vi "Bertta_v09_1.vi"() -> ()   [LabVIEW 2015]
panel:
  out "element":bool
  out "Started:":string
  in  "SHUTDOWN":bool
  in  "MASTER CONTROL":bool
  in  "Tab Control":T1(tab)
  in  "Read Seq":bool
  in  "Save Seq":bool
  in  "Configuration file":path=path "C:/Users/shresplab/Desktop/BerttaConfiguration.lvm" caption="Filename"
  in  "OK Button 2":bool
  out "Boolean":bool
  in  "User (initials)":string
  in  "Project name":string
  in  "Description":string
  out "Output file":string
  out "Sensor OK 6":bool
  out "Sensor OK 5":bool
  out "Sensor OK 4":bool
  out "Sensor OK 3":bool
  in  "OK Button":bool
  in  "Add comment":string
  out "PUMP 1":bool
  out "Target amount":dbl
  out "Scale weight":dbl
  out "Amount now":dbl
  out "Flow rate":dbl
  out "Time to target":dbl format="%<%H:%M:%S>t"
  out "Current step":dbl
  out "Target amount":dbl
  out "Amount now":dbl
  out "Tr":dbl
  out "Tj in":dbl
  out "Tj out":dbl
  out "T set":dbl
  out "Current step":i32
  out "RPM":dbl
  out "Torque 2":dbl
  out "Waveform Chart 5":dynamicdata(graph)
  out "Waveform Chart 6":dynamicdata(graph)
  out "Waveform Chart 7":dynamicdata(graph)
  out "Amount now":dbl
  out "Target amount":dbl
  out "Current step":dbl
  out "Time to target":dbl format="%<%H:%M:%S>t"
  out "Flow rate":dbl
  out "Amount now":dbl
  out "Scale weight":dbl
  out "Target amount":dbl
  out "PUMP 2":bool
  in  "Tab Control 2":T2(tab)
  out "Waveform Chart 3":dynamicdata(graph)
  out "Waveform Chart 8":dynamicdata(graph)
  out "Waveform Chart 11":dynamicdata(graph)
  out "Waveform Chart 9":dynamicdata(graph)
  out "Table":string[][](table)=[["14.8.2017 18.06.59", "0,000000", "417,670000", "-0,150000", "1,000000", "22,220000", "23,366837", "23,574959", "23,985852", "23,690000", "240,000000", "4,000000", "0,000000", "397,000000", "-397,000000", "1,000000"], ["14.8.2017 18.07.06", "0,000000", "417,640000", "-0,120000", "1,000000", "22,220000", "23,763115", "23,906257", "23,985694", "23,680000", "240,000000", "4,000000", "0,000000", "397,000000", "-397,000000", "1,000000"], ["14.8.2017 18.07.13", "0,000000", "417,640000", "-0,120000", "1,000000", "22,220000", "23,965922", "24,013440", "23,984906", "23,670000", "240,000000", "4,100000", "3,000000", "397,000000", "-397,000000", "1,000000"], ["14.8.2017 18.07.21", "0,000000", "417,640000", "-0,120000", "1,000000", "22,220000", "23,943860", "23,900110", "23,987113", "23,670000", "240,000000", "4,000000", "0,000000", "397,000000", "-397,000000", "1,000000"], ["14.8.2017 18.07.28", "0,000000", "417,640000", "-0,120000", "1,000000", "22,220000", "23,736328", "23,600018", "23,989004", "23,660000", "240,000000", "4,000000", "0,000000", "397,000000", "-397,000000", "1,000000"], ["14.8.2017 18.07.36", "0,000000", "417,640000", "-0,120000", "1,000000", "22,220000", "23,480910", "23,324538", "23,991053", "23,660000", "240,000000", "4,000000", "0,000000", "397,000000", "-397,000000", "1,000000"], ["14.8.2017 18.07.43", "0,000000", "417,640000", "-0,120000", "2,000000", "22,220000", "23,195579", "23,008270", "23,999093", "23,650000", "240,000000", "4,000000", "0,000000", "397,000000", "-397,000000", "1,000000"], ["14.8.2017 18.07.51", "0,000000", "417,650000", "-417,650000", "1,000000", "22,220000", "22,862541", "22,649021", "24,003979", "23,650000", "240,000000", "4,000000", "0,000000", "397,000000", "-397,000000", "2,000000"], ["14.8.2017 18.07.58", "0,000000", "417,640000", "0,010000", "1,000000", "22,220000", "22,541353", "22,354878", "24,005398", "23,650000", "240,000000", "4,000000", "0,000000", "397,000000", "-397,000000", "1,000000"], ["14.8.2017 18.08.06", "0,000000", "417,640000", "0,010000", "1,000000", "22,220000", "22,347931", "22,253738", "24,007605", "23,640000", "240,000000", "4,100000", "0,000000", "397,000000", "-397,000000", "1,000000"], ["14.8.2017 18.08.13", "0,000000", "417,640000", "0,010000", "1,000000", "22,220000", "22,329030", "22,302102", "24,006028", "23,640000", "240,000000", "4,000000", "0,000000", "395,820000", "-395,820000", "1,000000"], ["14.8.2017 18.08.20", "0,000000", "417,640000", "0,010000", "1,000000", "22,220000", "22,466849", "22,511320", "24,002403", "23,630000", "240,000000", "4,000000", "0,000000", "395,830000", "-0,010000", "1,000000"], ["14.8.2017 18.08.28", "0,000000", "417,640000", "0,010000", "1,000000", "22,220000", "22,707062", "22,835101", "24,000984", "23,620000", "240,000000", "4,000000", "0,000000", "395,830000", "-0,010000", "1,000000"], ["14.8.2017 18.08.35", "0,000000", "417,640000", "0,010000", "1,000000", "22,220000", "23,054104", "23,232979", "24,001299", "23,600000", "240,000000", "4,000000", "0,000000", "395,830000", "-0,010000", "1,000000"], ["14.8.2017 18.08.43", "0,000000", "417,640000", "0,010000", "1,000000", "22,220000", "23,412371", "23,522793", "24,002560", "23,590000", "240,000000", "4,000000", "0,000000", "395,820000", "0,000000", "1,000000"], ["14.8.2017 18.08.51", "0,000000", "417,640000", "0,010000", "1,000000", "22,220000", "23,596247", "23,656125", "24,003821", "23,580000", "240,000000", "4,000000", "0,000000", "395,820000", "0,000000", "1,000000"]]
  in  "T ext / T ext 2":enum32{"External 1", "External 2"}(radio)
  out "Sensor OK":bool
  in  "T fail":dbl=20.0
  out "Boolean 12":bool
  out "Boolean 7":bool
  out "Boolean 6":bool
  out "Boolean 5":bool
  out "Boolean 4":bool
  in  "?":bool
  in  "T manual setpoint":dbl=20.0
  in  "Lauda port":dbl=9.0
  in  "Manual select":enum32{"Tr", "Tj"}(radio)
  in  "TempSeq":dbl[][](array[numeric])=[[20.0, 40.0, 1.0, 30.0], [40.0, 50.0, 1.0, 30.0], [50.0, 20.0, 1.0, 30.0], [20.0, 20.0, 0.0, 20.0], [20.0, 20.0, 0.0, 20.0], [20.0, 20.0, 1000.0, 20.0]]
  out "T control":dbl
  out "Tr":dbl
  out "Tj in":dbl
  out "Tj out":dbl
  out "DT":dbl
  out "Elapsed":i32 format="%<%H:%M:%S>T"
  in  "PAUSE":bool
  out "Boolean 19":bool
  in  "Reset":bool
  in  "Treshold (Tset)":dbl=1.0
  in  "Tmax":dbl=199.0
  in  "Tmin":dbl=20.0
  out "Waveform Chart":dynamicdata(graph)
  out "T external 2":dbl
  in  "Xe":dbl=1.0
  in  "Ring":u16(ring) items=["SCALE 1", "SCALE 2", "SCALE 3"]
  out "Port":i32=10
  in  "Radio Buttons":enum32{"Reglo Digital", "Reglo Analog", "PAM"}(radio)=enum."Reglo Analog"
  out "Speed":dbl
  out "mA":dbl format="%#_2g"
  in  "Port":i32=14
  out "RPM":dbl format="%#_2g"
  out "Led10":bool
  out "Led9":bool
  out "Led8":bool
  out "Led7":bool
  out "Led6":bool
  out "Led5":bool
  out "Led4":bool
  out "Led3":bool
  out "Led2":bool
  out "Led1":bool
  in  "PumpSeq":dbl[][](array[numeric])=[[3.0, 3.0, 7.0], [2.0, 2.0, 2.0], [4.0, 2.0, 100.0], [0.0, 0.0, 0.0], [0.0, 0.0, 0.0], [0.0, 0.0, 0.0], [0.0, 0.0, 0.0], [0.0, 0.0, 0.0], [0.0, 0.0, 0.0], [0.0, 0.0, 0.0], [0.0, 1.0, 0.0]]
  in  "?":bool
  out "Flow rate (g/min)":dbl
  out "Scale reading":dbl
  out "Step amount now":dbl
  out "Time to target":dbl format="%<%H:%M:%S>t"
  in  "Grams / min":dbl
  out "Waveform Chart 2":dynamicdata(graph)
  in  "?":bool
  out "Total amount now":dbl
  out "Total time":dbl
  out "Total amount target":dbl
  out "Led11":bool
  in  "Reset 2":bool
  in  "Bypass select 2":enum32{"Remote", "Manual"}(radio)
  in  "Port":dbl=13.0
  out "RPM":dbl
  out "Torque":dbl
  in  "Set RPM":dbl(slide) scale=0.0..500.0
  out "Waveform Chart 4":dynamicdata(graph)
  out "DAQ 9217 (PT100)":errorcluster
  # "PUMP & SCALE 1"
  # "PUMP & SCALE 2"
  # "STEP"
  # "STEP"
  # "TOTAL"
  # "TOTAL"
  # "Temperature sensor:"
  # "Manual control:"
  # "Tinit     >    Tset       Min. time      Tfail"
  # "Manual control / end of sequence"
  # "Manual control"
  # "Secondary temperature sensor"
  # "Device communication"
  # "Grams    /   min"
  # "End of sequence"
  # "Manual control"
  # "Device communication"
  # "Pump configuration"
  # "Scale configuration"
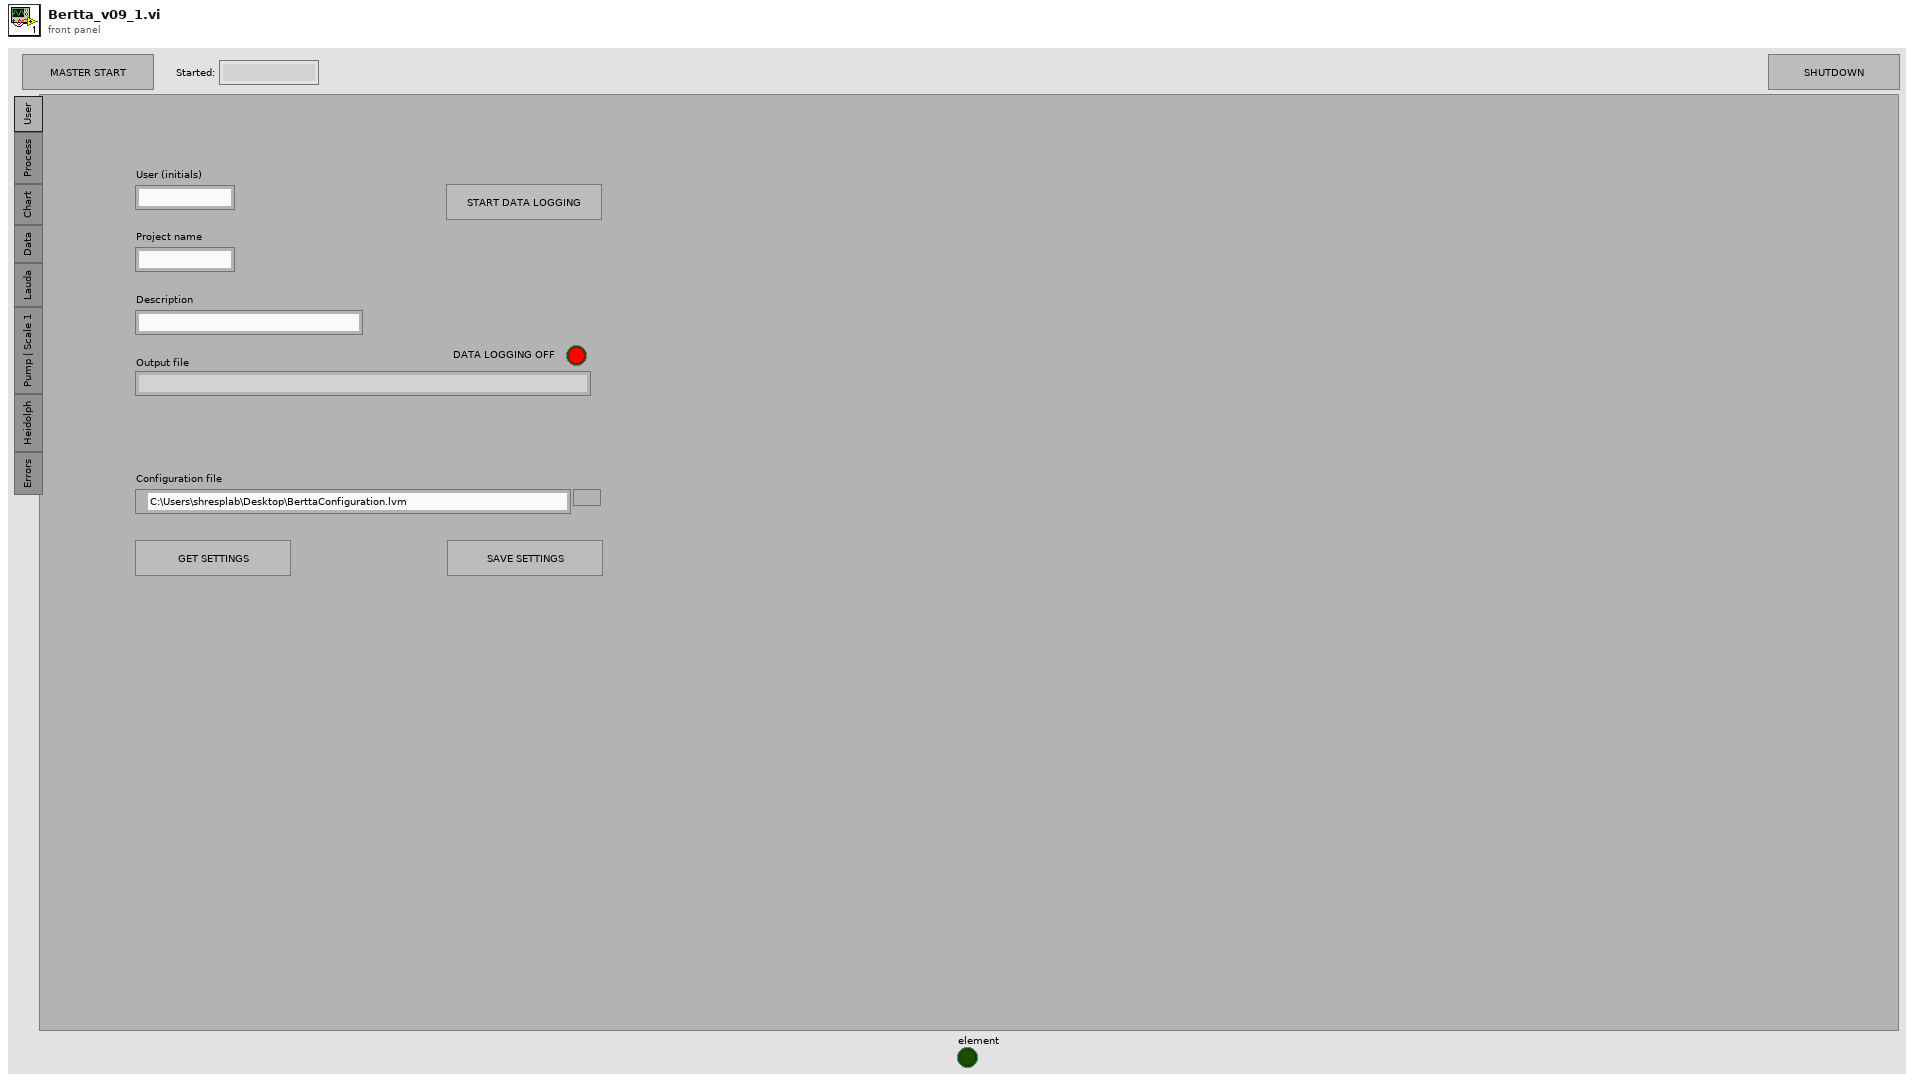
[diagram p1: front panel]
types:
  T1 = enum32{"User", "Process", "Chart", "Data", "Lauda", "Pump | Scale 1", "Heidolph", "Errors"}
  T2 = enum32{"Temperatures", "Scale / Pump 1", "Scale / Pump 2", "RPM / torque"}
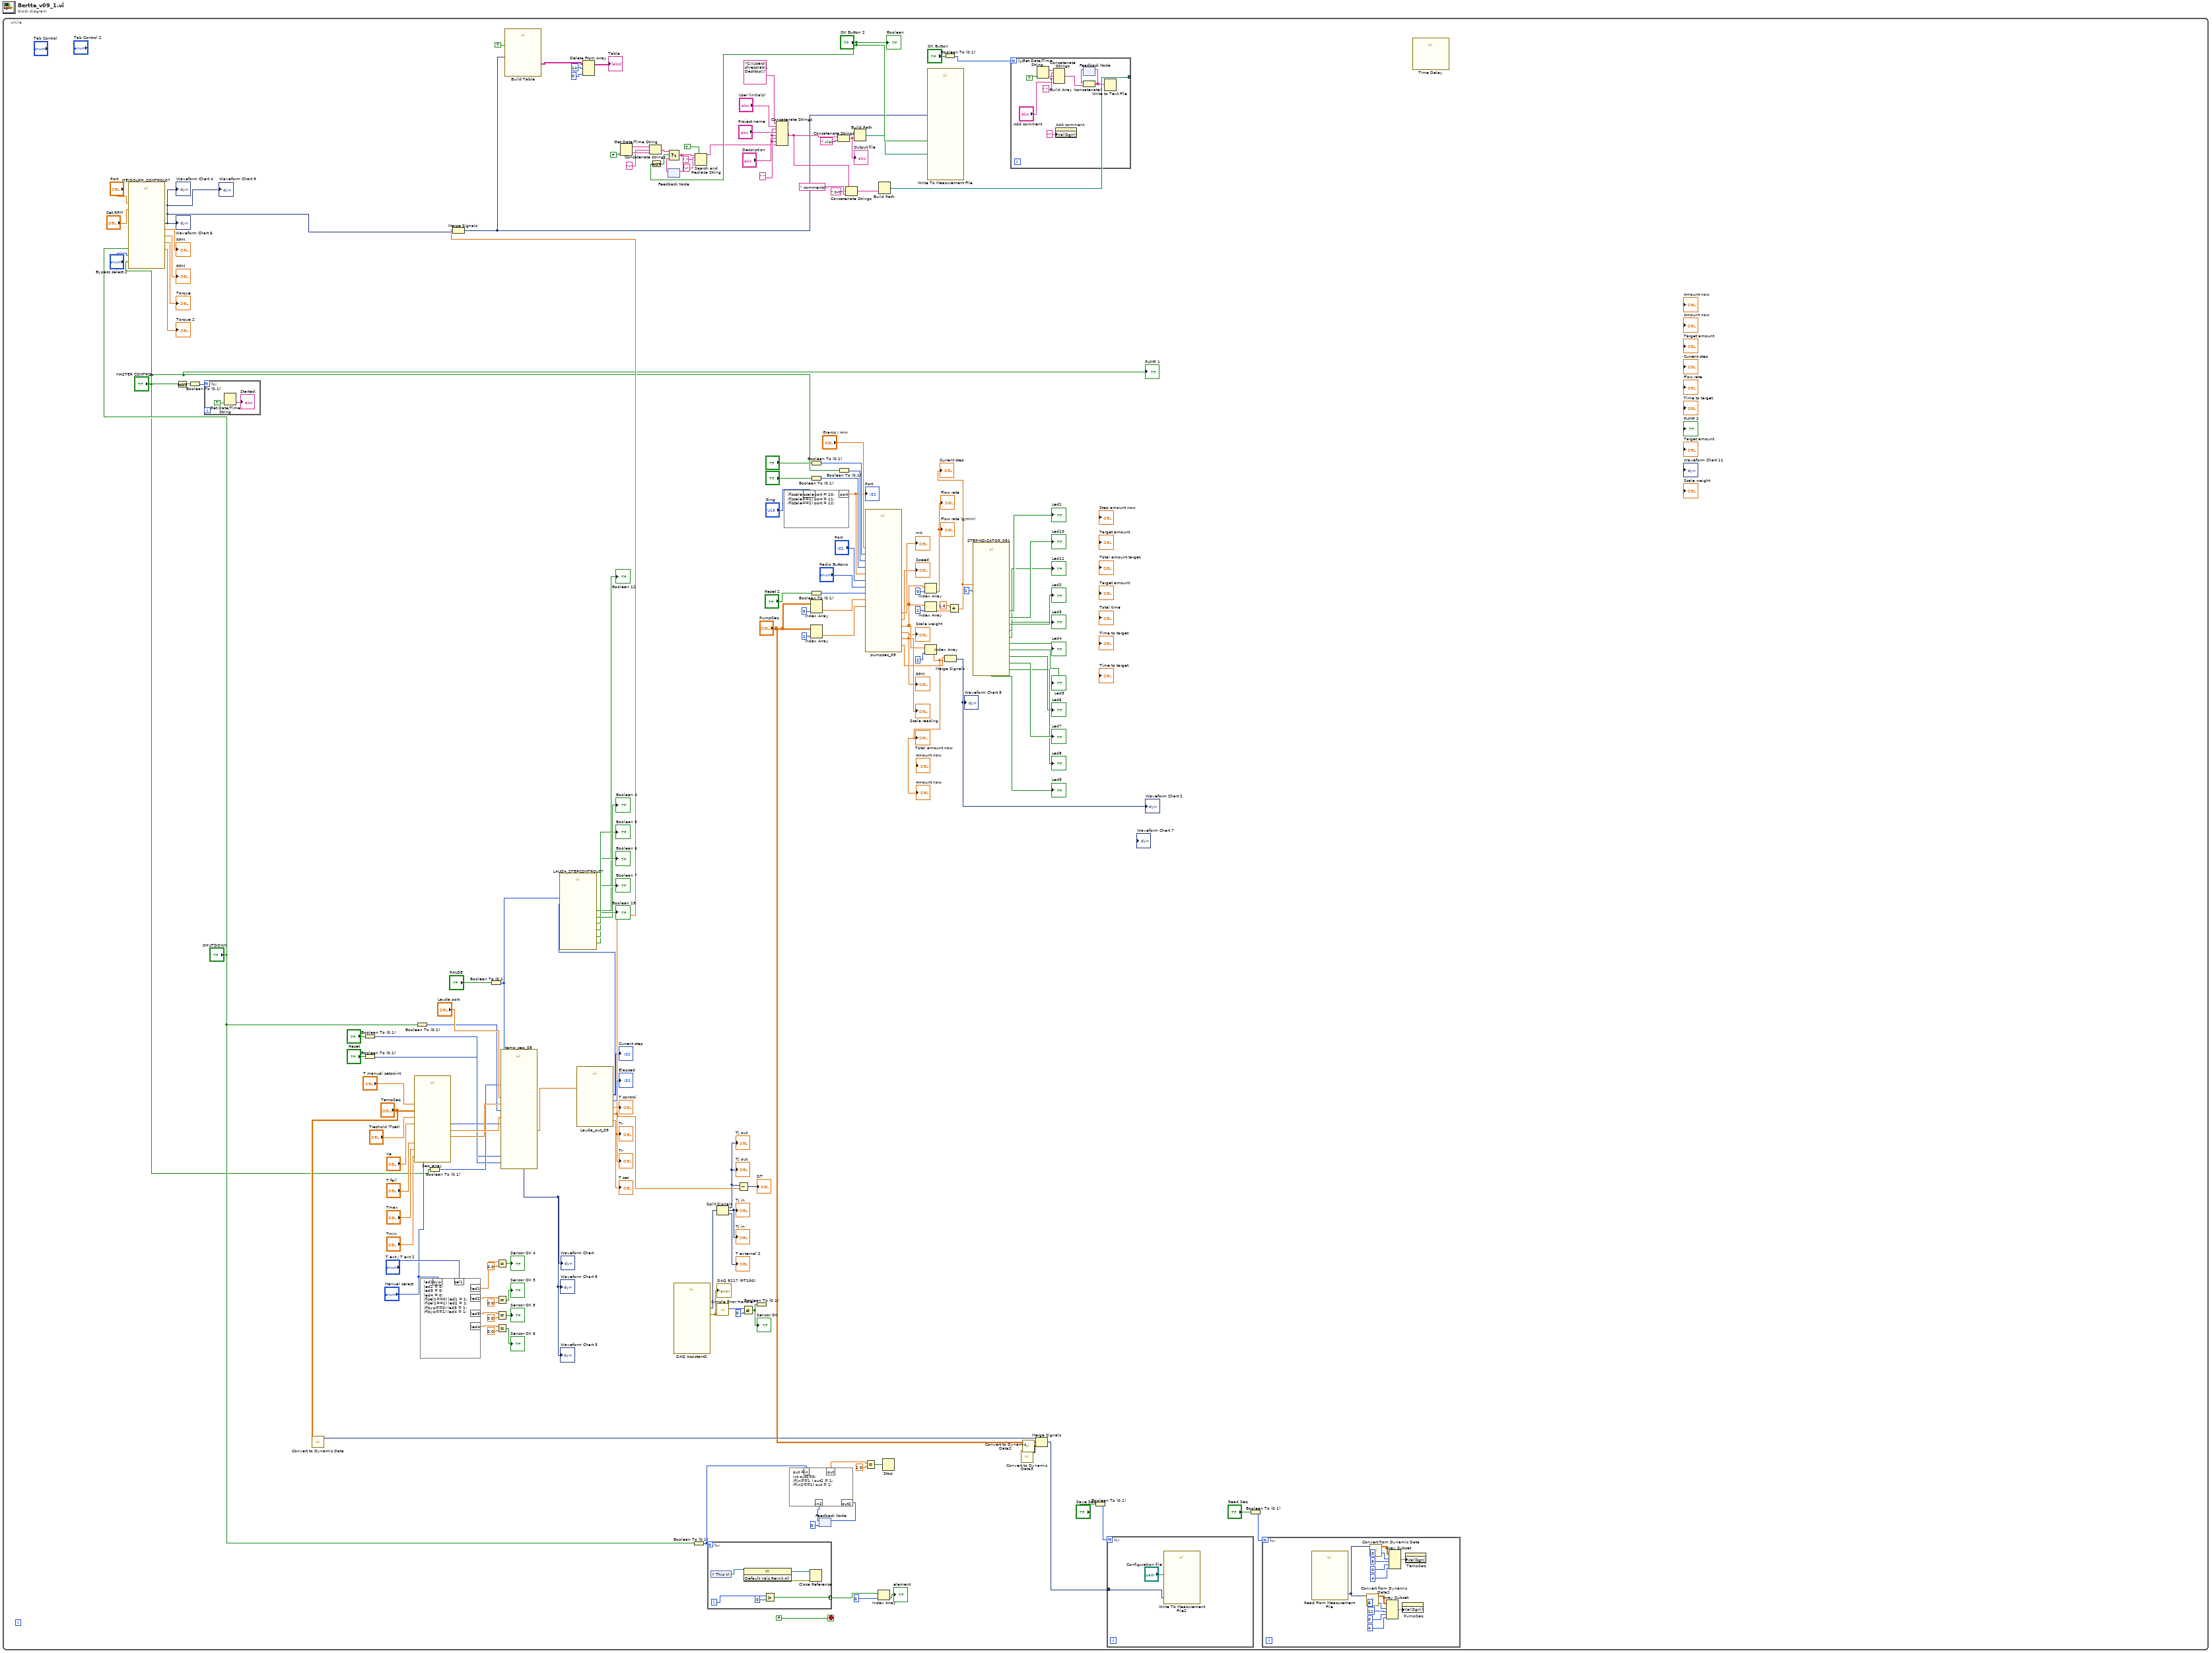
[diagram p0: block diagram]
diagram:
  n1 = while {
    stop <- FALSE stop-if-true
    w146 = " "
    n2 = call "HEIDOLPH_CONTROL07.vi"("master"="MASTER CONTROL", "shutdown"="SHUTDOWN", "Bypass select"="Bypass select 2", "Set RPM"="Set RPM", "Device port"="Port") -> ("Dynamic Data"=w157:dynamicdata, "RPM"=→"RPM":dbl, "RPM 2"=→"RPM":dbl, "Torque"=→"Torque":dbl, "Torque 2"=→"Torque 2":dbl)  [unwired: 2 in]
    "Waveform Chart 4" <- w157
    "Waveform Chart 6" <- w157
    "Waveform Chart 9" <- w157
    n3 = Not(x="MASTER CONTROL") -> (.not. x?=w139:bool)
    n4 = Boolean To (0,1)(Boolean=w139) -> (0, 1=w140:i16)
    n5 = for {
      N: w140 -> [_]
      n6 = Get Date/Time String(want seconds? (F)=TRUE) -> (time string=→"Started:":string)  [unwired: 2 in, 1 out]
    }
    n7 = call "Convert to Dynamic Data"("2D Array"="TempSeq") -> ("Dynamic Data Type"=w136:dynamicdata)  [unwired: 3 in]
    n8 = Boolean To (0,1)(Boolean="Reset") -> (0, 1=w58:i16)
    n9 = Boolean To (0,1)(Boolean="?") -> (0, 1=w60:i16)
    n10 = call "Seq_array.vi"("Tfail_manual"="T fail", "TempSeq in"="TempSeq", "Tmin"="Tmin", "Tmax"="Tmax", "Treshold (Tset)"="Treshold (Tset)", "T manual setpoint"="T manual setpoint", "Xe"="Xe") -> ("TimeParams"=w73:dbl[], "TempParams"=w74:dbl[])  [unwired: 3 in]
    n11 = Boolean To (0,1)(Boolean="SHUTDOWN") -> (0, 1=w69:i16)
    n12 = formula code="led1 = 0;\nled2 = 0;\nled3 = 0;\nled4 = 0;\nif(sel1==0) led1 = 1;\nif(sel1==1) led2 = 1;\nif(byp==0) led3 = 1;\nif(byp==1) led4 = 1;"("sel1"="T ext / T ext 2", "byp"="Manual select") -> ("led1"=w89:dbl, "led2"=w87:dbl, "led3"=w82:dbl, "led4"=w81:dbl)
    n13 = Boolean To (0,1)(Boolean="MASTER CONTROL") -> (0, 1=w68:i16)
    n14 = Boolean To (0,1)(Boolean="PAUSE") -> (0, 1=w64:i16)
    n15 = Equal?(x=w89, y=0.0) -> (x = y?=→"Sensor OK 4":bool)
    n16 = Equal?(x=w87, y=0.0) -> (x = y?=→"Sensor OK 3":bool)
    n17 = Equal?(x=w82, y=0.0) -> (x = y?=→"Sensor OK 5":bool)
    n18 = Equal?(x=w81, y=0.0) -> (x = y?=→"Sensor OK 6":bool)
    n19 = call "temp_seq_09.vi"("master"=w68, "shutdown"=w69, "Tr_orTj"="Manual select", "pause"=w64, "TempParams"=w74, "TimeParams"=w73, "port"="Lauda port", "reset"=w58, "manual"=w60) -> ("params"=w66:dbl[], "Waveform Chart"=→"Waveform Chart 3" →"Waveform Chart" →"Waveform Chart 5":dynamicdata)  [unwired: 3 in, 2 out]
    n20 = call "Lauda_out_09.vi"("params"=w66) -> ("Elapsed"=→"Elapsed":i32, "Tr"=w48:dbl, "Current step"=w47:i32, "T control"=→"T control":dbl, "T set"=→"T set":dbl)  [unwired: 6 in]
    "Tr" <- w48
    "Tr" <- w48
    "Current step" <- w47
    n21 = Merge Signals(w48, w157) -> (w112:dynamicdata)
    n22 = call "Build Table"("Include time data"=TRUE, "Signals"=w112) -> ("Table"=w111:string[][])  [unwired: 3 in, 6 out]
    n23 = call "LAUDA_STEPCONTROL07.vi"("step"=w47, "pause"=w64) -> ("Boolean 13"=→"Boolean 19":bool, "Boolean 6"=→"Boolean 6":bool, "Boolean 5"=→"Boolean 5":bool, "Boolean 4"=→"Boolean 4":bool, "Boolean 7"=→"Boolean 7":bool, "Boolean 12"=→"Boolean 12":bool)  [unwired: 4 in]
    n24 = Delete From Array(array=w111, length=14, index (col)=0 ("index (row)")) -> (array with subset deleted=→"Table":string[][])  [unwired: 1 in, 1 out]
    n25 = Get Date/Time String(want seconds? (F)=FALSE) -> (date string=w125:string, time string=w120:string)  [unwired: 2 in]
    n26 = Concatenate Strings(w125, "-" ("string"), w120) -> (w124:string)
    n27 = Not(x="OK Button 2") -> (.not. x?=w121:bool)
    n28 = feedback #1() -> (w123:string)  [unwired: 1 in]
    n29 = Select(t=w124, s=w121, f=w123) -> (s? t:f=w116:string)
    n30 = feedback-in #1(w116) -> ()
    n31 = call "DAQ Assistant2"() -> ("data"=w53:dynamicdata, "error out"=w152:errorcluster)  [unwired: 17 in, 1 out]
    "DAQ 9217 (PT100)" <- w152
    n32 = Boolean To (0,1)(Boolean="SHUTDOWN") -> (0, 1=w95:i16)
    n33 = Search and Replace String(replace all?=TRUE ("replace all? (F)"), input string=w116, search string=".", replace string="-" ("replace string (\"\")")) -> (result string=w115:string)  [unwired: 4 in, 3 out]
    n34 = for {
      N: w95 -> [_]
      tunnel: [w189] -> w138 mode=indexing
      i -> [w191]
      n35 = control-ref of="This VI"() -> (w194:refnum<vi>)
      n36 = invoke class="VI" method="Default Vals.Reinit All"(reference=w194) -> (reference out=w192:refnum<vi>, error out=w193:errorcluster)  [unwired: 2 in, 1 out]
      n37 = Greater?(x=w191, y=0) -> (0:w189:bool)
      n38 = Close Reference(reference=w192, error in (no error)=w193) -> ()  [unwired: 1 out]
    }
    n39 = Split Signals(w53) -> (w50:dynamicdata, →"Tj in" →"Tj in":dynamicdata, →"T external 2":dynamicdata)  [unwired: 3 in]
    "Tj out" <- w50
    "Tj out" <- w50
    n40 = call <vilib>:"Simple Error Handler.vi"("error in (no error)"=w152) -> ("code out"=w151:i32)  [unwired: 4 in, 4 out]
    n41 = Subtract(x=w50, y=w48) -> (x-y=→"DT":dynamicdata)
    n42 = Not Equal?(x=w151, y=0) -> (x != y?=w129:bool)
    "Sensor OK" <- w129
    n43 = Boolean To (0,1)(Boolean=w129) -> ()  [unwired: 1 out]
    n44 = Concatenate Strings("C:\\Users\\shresplab\\Desktop\\", "User (initials)", w146, "Project name", w146, "Description", w146, w115) -> (w105:string)
    n45 = formula code="if(scale==0) port = 10;\nif(scale==1) port = 11;\nif(scale==2) port = 12;"("scale"="Ring") -> ("port"=w28:dbl)
    "Port" <- w28
    n46 = Boolean To (0,1)(Boolean="?") -> (0, 1=w38:i16)
    n47 = Boolean To (0,1)(Boolean="?") -> (0, 1=w34:i16)
    n48 = Boolean To (0,1)(Boolean="Reset 2") -> (0, 1=w36:i16)
    n49 = Index Array(array="PumpSeq", index (col)=0 ("disabled index (col)")) -> (element=w43:dbl[])  [unwired: 1 in]
    n50 = Index Array(array="PumpSeq", index (col)=1 ("disabled index (col)")) -> (element=w42:dbl[])  [unwired: 1 in]
    n51 = feedback #2(0) -> (w93:i32)
    n52 = formula code="out = 0;\nint out2=0;\nif(in==1 ) out2 = 1;\nif(in2==1) out = 1;"("in"=w95, "in2"=w93) -> ("out"=w97:dbl, "out2"=w94:i32)
    n53 = feedback-in #2(w94) -> ()
    n54 = Concatenate Strings(w105, ".xlsx") -> (w108:string)
    "Output file" <- w108
    n55 = Boolean To (0,1)(Boolean="MASTER CONTROL") -> (0, 1=w32:i16)
    n56 = Concatenate Strings(w105, " comments" ("string"), ".txt" ("string")) -> (w102:string)
    n57 = Build Path(name or relative path=w108) -> (appended path=w106:path)  [unwired: 1 in]
    n58 = Equal?(x=w97, y=1.0) -> (x = y?=w96:bool)
    n59 = call "pumpsec_09.vi"("reset"=w36, "pump_type"="Radio Buttons", "Target"=w43, "fr_manual"="Grams / min", "master"=w32, "manual"=w38, "pause"=w34, "Port"=w28, "port, Reglo D"="Port", "Time"=w42) -> ("Scale"=→"Scale reading" →"Scale weight":dbl, "mA"=→"mA":dbl, "Scale actual"=w4:dbl, "params"=w22:dbl[], "Reglo D"=→"RPM":dbl, "PAM"=→"Speed":dbl)
    n60 = Index Array(array=w138, index=0) -> (element=→"element":bool)
    n61 = Build Path(name or relative path=w102) -> (appended path=w101:path)  [unwired: 1 in]
    n62 = Stop(stop? (T)=w96) -> ()
    n63 = Index Array(array=w22, index=0) -> (element=→"Flow rate (g/min)" →"Flow rate":dbl)
    n64 = Index Array(array=w22, index=1) -> (element=w24:dbl)
    n65 = Index Array(array=w22, index=2) -> (element=w2:dbl)
    "Total amount now" <- w2
    "Amount now" <- w2
    n66 = call "Write To Measurement File"("Signals"=w112, "Enable"="OK Button 2", "Filename"=w106) -> ()  [unwired: 14 in, 3 out]
    n67 = Boolean To (0,1)(Boolean="OK Button") -> (0, 1=w100:i16)
    n68 = Merge Signals(w4, w2) -> (→"Waveform Chart 2" →"Waveform Chart 8":dynamicdata)
    n69 = Add(x=1.0, y=w24) -> (x+y=w5:dbl)
    "Current step" <- w5
    n70 = call "STEPINDICATOR_091.vi"("current step"=w5, "enable"=i16 1) -> ("Led 8"=→"Led8":bool, "Led 10"=→"Led10":bool, "Led 11"=→"Led11":bool, "Led 7"=→"Led7":bool, "Led 1"=→"Led1":bool, "Led 6"=→"Led6":bool, "Led 2"=→"Led2":bool, "Led 5"=→"Led5":bool, "Led 4"=→"Led4":bool, "Led 3"=→"Led3":bool, "Led 9"=→"Led9":bool)  [unwired: 3 in]
    n71 = for {
      N: w100 -> [_]
      tunnel: w101 -> [w166]
      w170 = " " ("string")
      n72 = Get Date/Time String(want seconds? (F)=TRUE) -> (date string=w173:string, time string=w171:string)  [unwired: 2 in]
      n73 = Concatenate Strings(w173, w170, w171, w170, "Add comment") -> (w169:string)
      n74 = property on="Add comment" class="Str"("Val(Sgnl)"="" ("Value (Signaling)")) -> ()  [unwired: 2 in, 2 out]
      n75 = feedback #3() -> (w168:string[])  [unwired: 1 in]
      n76 = Build Array (concatenate)(w168, w169) -> (w167:string[])
      n77 = feedback-in #3(w167) -> ()
      n78 = Write to Text File(file (use dialog)=w166, text=w167) -> ()  [unwired: 2 in, 3 out]
    }
    n79 = call "Convert to Dynamic Data3"() -> ("Dynamic Data Type"=w78:dynamicdata)  [unwired: 4 in]
    n80 = call "Convert to Dynamic Data2"("2D Array"="PumpSeq") -> ("Dynamic Data Type"=w135:dynamicdata)  [unwired: 3 in]
    n81 = Merge Signals(w136, w135, w78) -> (w134:dynamicdata)
    n82 = Boolean To (0,1)(Boolean="Save Seq") -> (0, 1=w133:i16)
    n83 = for {
      N: w133 -> [_]
      tunnel: w134 -> [w188]
      n84 = call "Write To Measurement File2"("Signals"=w188, "Filename"="Configuration file") -> ()  [unwired: 15 in, 3 out]
    }
    n85 = Boolean To (0,1)(Boolean="Read Seq") -> (0, 1=w130:i16)
    n86 = for {
      N: w130 -> [_]
      n87 = call "Read From Measurement File"() -> ("Signals"=w176:dynamicdata)  [unwired: 6 in, 5 out]
      n88 = call "Convert from Dynamic Data2"("Dynamic Data Type"=w176) -> ("Array"=w175:dbl[][])  [unwired: 3 in]
      n89 = call "Convert from Dynamic Data"("Dynamic Data Type"=w176) -> ("Array"=w184:dbl[][])  [unwired: 3 in]
      n90 = Array Subset(array=w175, index (row)=6 ("index"), length (row)=11 ("length"), index (col)=0 ("index"), length (col)=4 ("length")) -> (w174:dbl[][])
      n91 = Array Subset(array=w184, index (row)=0 ("index"), length (row)=6 ("length"), index (col)=0 ("index"), length (col)=4 ("length")) -> (w181:dbl[][])
      n92 = property on="PumpSeq" class="Arr (strict)"("Val(Sgnl)"=w174) -> ()  [unwired: 2 in, 2 out]
      n93 = property on="TempSeq" class="Arr (strict)"("Val(Sgnl)"=w181) -> ()  [unwired: 2 in, 2 out]
    }
    n94 = call "Time Delay"() -> ()  [unwired: 11 in, 1 out]
    "PUMP 1" <- "MASTER CONTROL"
    "Boolean" <- "OK Button 2"
  }
